vi "traffic control lights IO.vi"(0 "red channels":string[](array[string]), 1 "state":u16(ring) items=["Init", "Write", "Read", "Close"], 2 "skred detektert av mast":bool[](array[boolean]), 3 "Mast vs skredløp output":u8[](array[numeric]), 9 "enable signallys":bool, 11 "error in":errorcluster) -> (6 "røde lys indikator":bool[][](array[boolean]), 15 "error out":errorcluster)   [LabVIEW 2017]
uses:
  <vilib>/DAQmx/write.llb/DAQmx Write (Digital 1D Bool NChan 1Samp 1Line).vi
  <vilib>/DAQmx/read.llb/DAQmx Read (Digital 1D Bool NChan 1Samp 1Line).vi
  <vilib>/DAQmx/create/channels.llb/DAQmx Create Channel (DO-Digital Output).vi
  <vilib>/DAQmx/miscellaneous.llb/DAQmx Fill In Error Info.vi
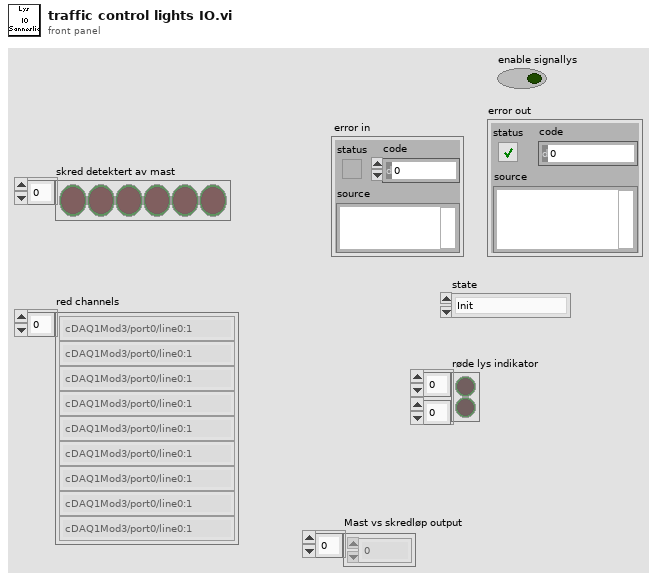
[diagram p1: front panel]
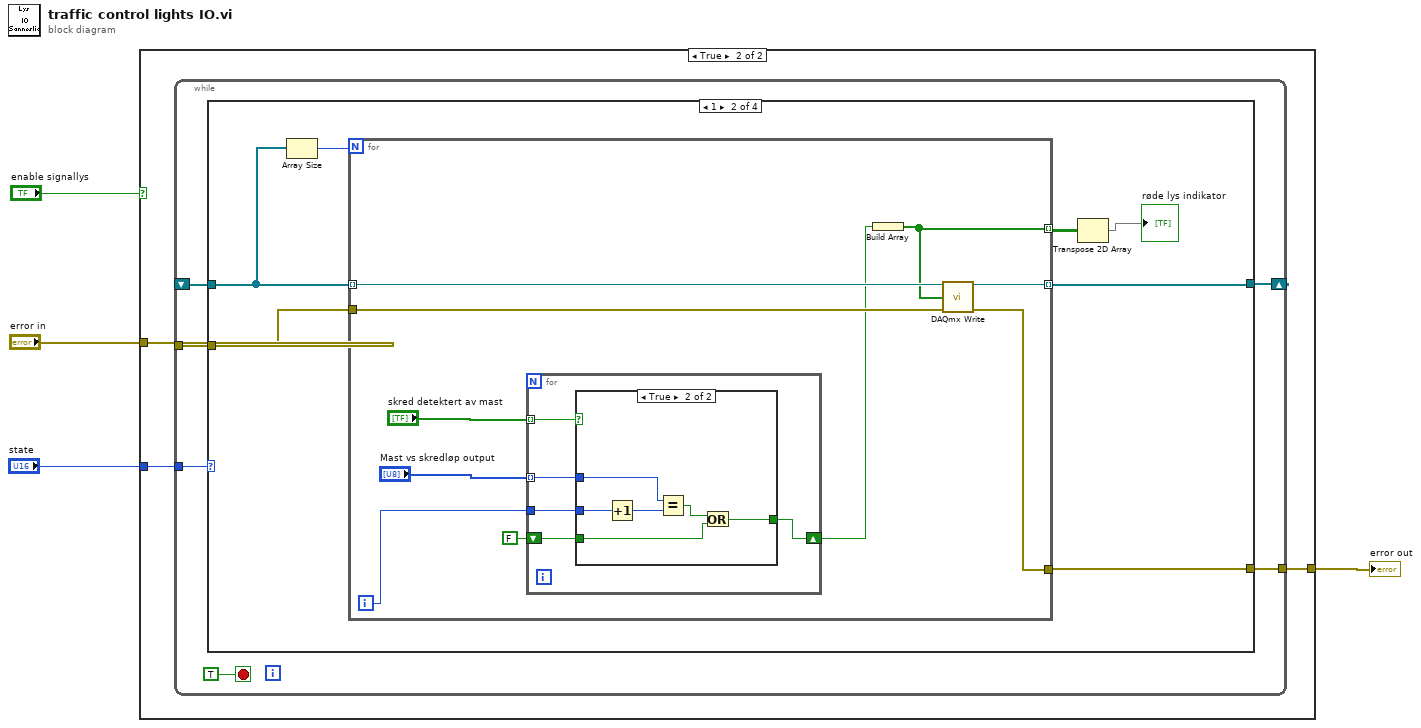
[diagram p0: block diagram]
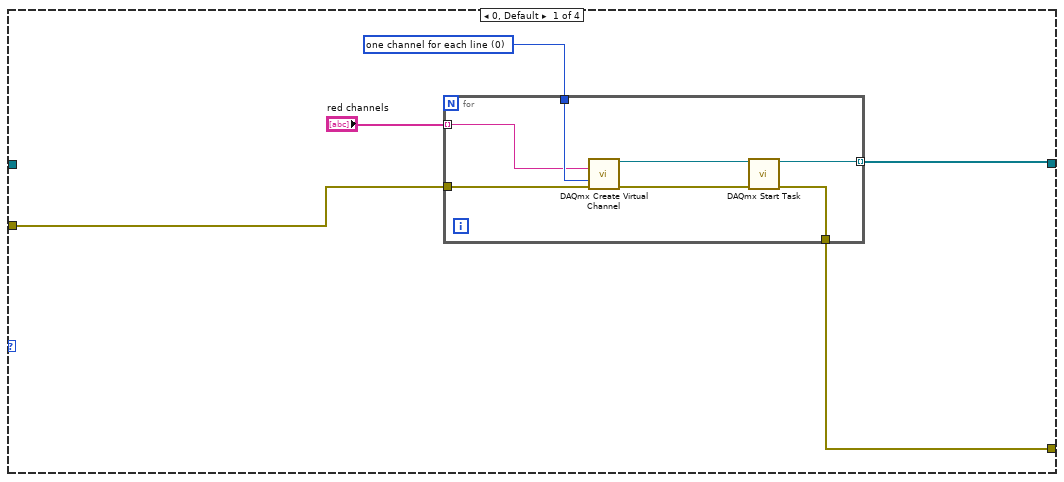
[diagram p3: hidden frame]
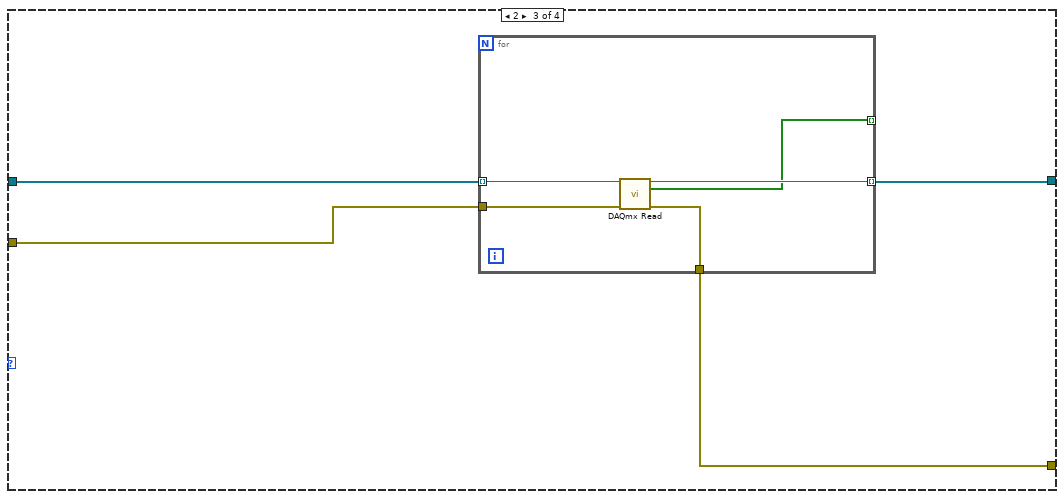
[diagram p5: hidden frame]
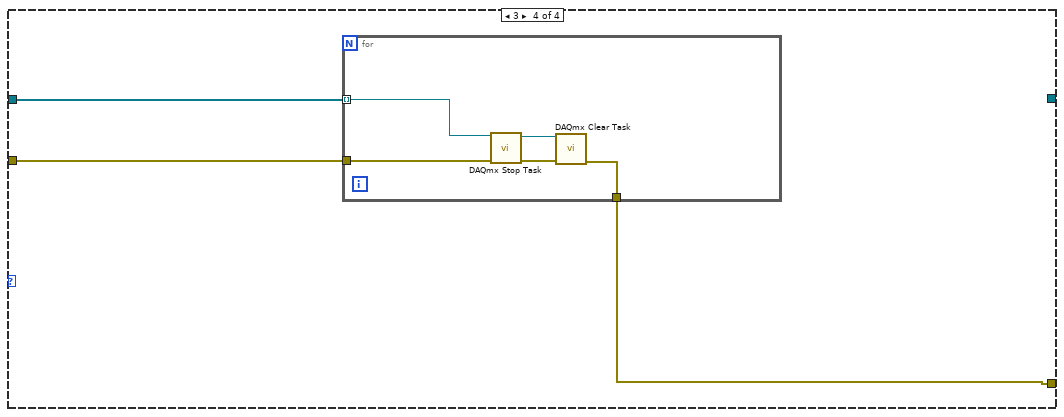
[diagram p6: hidden frame]
diagram:
  n1 = case shown="True" "enable signallys" {
    tunnel: "state" -> [_ w8]
    tunnel: "error in" -> [w5 w7]
    tunnel: [w5 w6] -> w2
    frame False {
    }
    frame True {
      n2 = while {
        tunnel: w8 -> [w9]
        shift-right: [w13] -> _
        shift-left: _ -> [w11]
        tunnel: w7 -> [w12]
        tunnel: [w10] -> w6
        stop <- TRUE stop-if-true
        n3 = case shown="1" w9 {
          tunnel: [w18 w32 w57 _] -> w13
          tunnel: [w15 w29 w56 w65] -> w10
          tunnel: w12 -> [w16 w33 w58 w67]
          tunnel: w11 -> [_ w30 w59 w66]
          frame 0, Default {
            w17 = 0 items=["one channel for each line", "one channel for all lines"] ("line grouping")
            n4 = for {
              tunnel: "red channels" -> [w20] mode=indexing
              tunnel: [w23] -> w18 mode=indexing
              tunnel: w17 -> [w26]
              tunnel: w16 -> [w25]
              tunnel: [w21] -> w15
              n5 = call-poly <vilib>:"DAQmx Create Virtual Channel.vi"("lines"=w20, "line grouping"=w26, "error in"=w25) -> ("task out"=w24:refnum<k21>, "error out"=w22:errorcluster)  [unwired: 11 in]
              n6 = call <vilib>:"DAQmx Start Task.vi"("task/channels in"=w24, "error in"=w22) -> ("task out"=w23:refnum<k21>, "error out"=w21:errorcluster)  [unwired: 12 in]
            }
          }
          frame 1 {
            n7 = Array Size(array=w30) -> (size(s)=w31:i32)
            n8 = for {
              N: w31 -> [_]
              tunnel: w30 -> [w43] mode=indexing
              tunnel: w33 -> [w42]
              tunnel: [w41] -> w29
              tunnel: [w40] -> w32 mode=indexing
              tunnel: [w34] -> w28 mode=indexing
              i -> [w37]
              n9 = for {
                tunnel: "skred detektert av mast" -> [w48] mode=indexing
                tunnel: "Mast vs skredløp output" -> [w46] mode=indexing
                tunnel: w37 -> [w47]
                shift-right: [w44] -> w35
                shift-left: FALSE -> [w45]
                n10 = case shown="True" w48 {
                  tunnel: w47 -> [_ w55]
                  tunnel: w46 -> [_ w53]
                  tunnel: w45 -> [w49 w51]
                  tunnel: [w49 w50] -> w44
                  frame False {
                  }
                  frame True {
                    n11 = Increment(x=w55) -> (x+1=w54:i32)
                    n12 = Equal?(x=w53, y=w54) -> (x = y?=w52:bool)
                    n13 = Or(x=w52, y=w51) -> (x .or. y?=w50:bool)
                  }
                }
              }
              n14 = Build Array(w35) -> (w34:bool[])
              n15 = call-poly <vilib>:"DAQmx Write.vi"("task/channels in"=w43, "data"=w34, "error in"=w42) -> ("task out"=w40:refnum<k21>, "error out"=w41:errorcluster)  [unwired: 10 in, 1 out]
            }
            n16 = Transpose 2D Array(2D array=w28) -> (transposed array=→"røde lys indikator":bool[][])
          }
          frame 2 {
            n17 = for {
              tunnel: w59 -> [w64] mode=indexing
              tunnel: w58 -> [w63]
              tunnel: [w62] -> w56
              tunnel: [w61] -> w57 mode=indexing
              tunnel: [w60] -> _ mode=indexing
              n18 = call-poly <vilib>:"DAQmx Read.vi"("task/channels in"=w64, "error in"=w63) -> ("task out"=w61:refnum<k21>, "data"=w60:bool[], "error out"=w62:errorcluster)  [unwired: 11 in]
            }
          }
          frame 3 {
            n19 = for {
              tunnel: w67 -> [w69]
              tunnel: w66 -> [w68] mode=indexing
              tunnel: [w72] -> w65
              n20 = call <vilib>:"DAQmx Stop Task.vi"("task/channels in"=w68, "error in"=w69) -> ("task out"=w71:refnum<k21>, "error out"=w70:errorcluster)  [unwired: 12 in]
              n21 = call <vilib>:"DAQmx Clear Task.vi"("task in"=w71, "error in"=w70) -> ("error out"=w72:errorcluster)  [unwired: 13 in]
            }
          }
        }
      }
    }
  }
  "error out" <- w2
